vi "字符串案例之字符串公式解析(下).vi"() -> ()   [LabVIEW 2018]
panel:
  out "数组 5":dbl[](array[numeric])
  out "数组 4":dbl[](array[numeric])
  out "数组 3":string[](array[string])
  out "数组 2":string[](array[string])
  out "数组":dbl[](array[numeric])
  in  "字符串":string
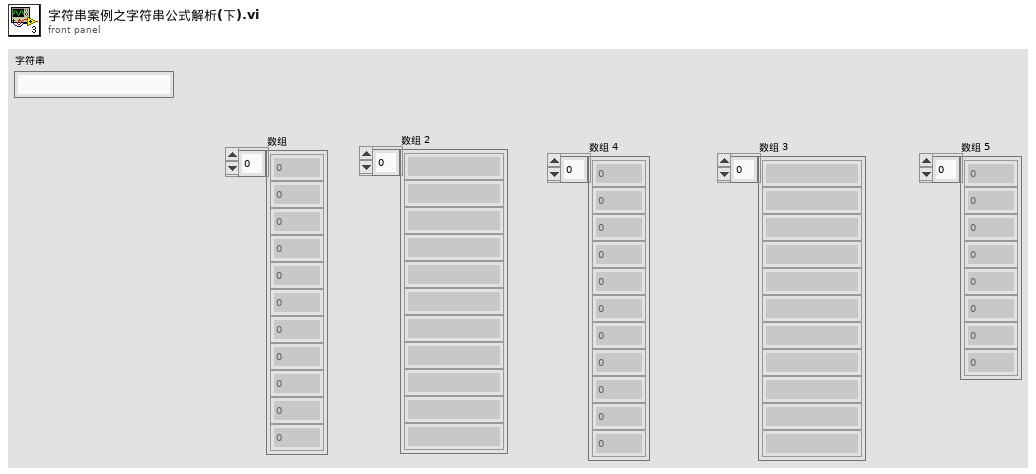
[diagram p1: front panel]
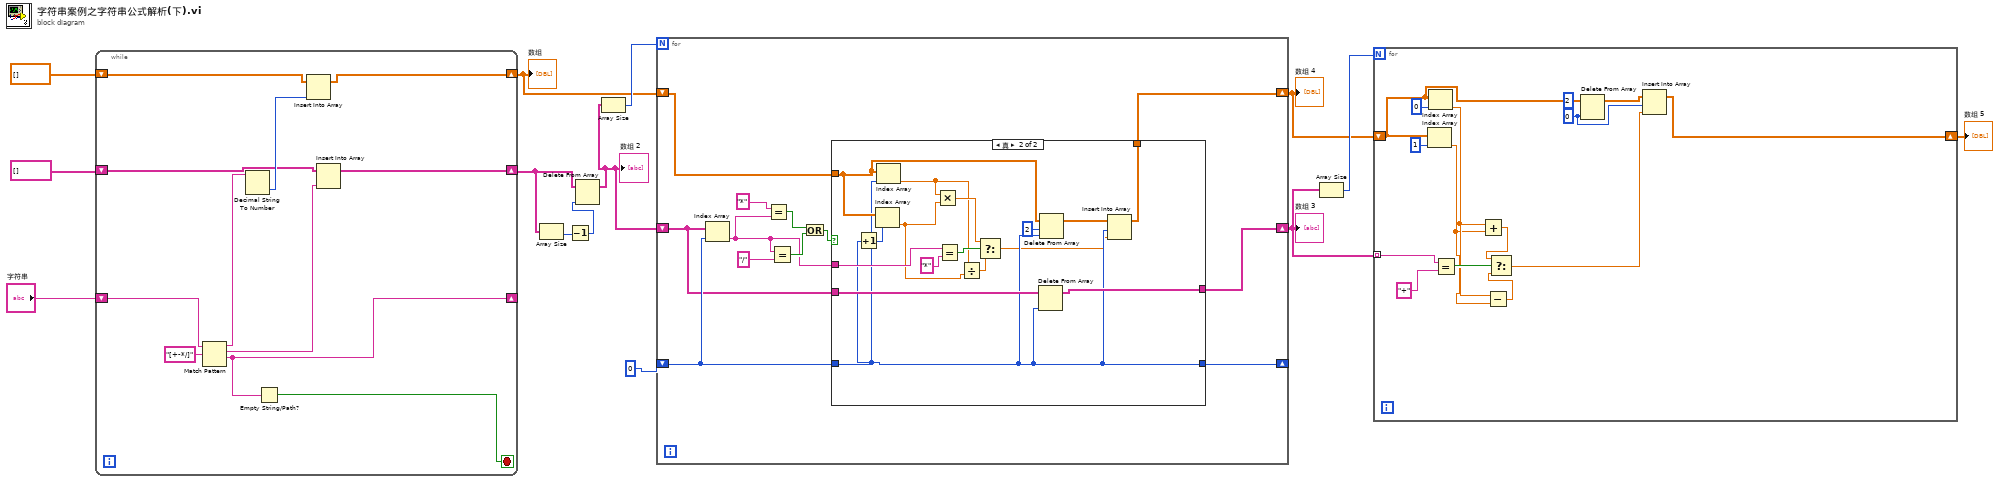
[diagram p0: block diagram]
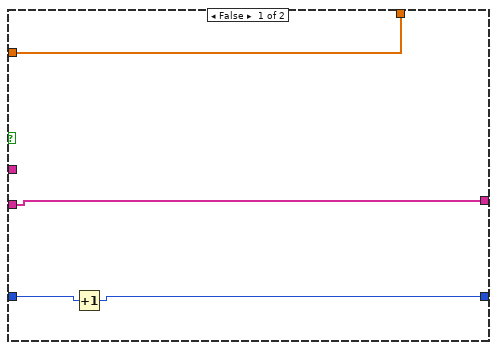
[diagram p2: hidden frame]
diagram:
  n1 = while {
    shift-right: [w20] -> w5
    shift-left: dbl[] [] -> [w21]
    shift-right: [w17] -> w11
    shift-left: string[] [] -> [w18]
    shift-right: [w16] -> _
    shift-left: "字符串" -> [w24]
    stop <- w15 stop-if-true
    n2 = Match Pattern(string=w24, regular expression="[+-*/]" ("正则表达式")) -> (before substring=w23:string, match substring=w19:string, after substring=w16:string)  [unwired: 1 in, 1 out]
    n3 = Decimal String To Number(string=w23) -> (number=w22:i32)  [unwired: 2 in, 1 out]
    n4 = Empty String/Path?(string/path=w16) -> (empty?=w15:bool)
    n5 = Insert Into Array(array=w21, new element=w22) -> (w20:dbl[])  [unwired: 1 in]
    n6 = Insert Into Array(array=w18, new element=w19) -> (w17:string[])  [unwired: 1 in]
  }
  "数组" <- w5
  n7 = Array Size(array=w11) -> (size(s)=w10:i32)
  n8 = Decrement(x=w10) -> (x-1=w9:i32)
  n9 = Delete From Array(array=w11, index=w9) -> (array with subset deleted=w7:string[])  [unwired: 1 in, 1 out]
  "数组 2" <- w7
  n10 = Array Size(array=w7) -> (size(s)=w8:i32)
  n11 = for {
    N: w8 -> [_]
    shift-right: [w32] -> _
    shift-left: 0 -> [w31]
    shift-right: [w29] -> w3
    shift-left: w7 -> [w30]
    shift-right: [w26] -> w2
    shift-left: w5 -> [w28]
    n12 = Index Array(array=w30, index=w31) -> (element=w27:string)
    n13 = Equal?(x="*", y=w27) -> (x = y?=w34:bool)
    n14 = Equal?(x=w27, y="/") -> (x = y?=w35:bool)
    n15 = Or(x=w34, y=w35) -> (x .or. y?=w33:bool)
    n16 = case shown="真" w33 {
      tunnel: w31 -> [w41 w44]
      tunnel: [w40 w44] -> w32
      tunnel: w30 -> [w39 w57]
      tunnel: [w39 w56] -> w29
      tunnel: w28 -> [w38 w47]
      tunnel: w27 -> [_ w53]
      tunnel: [w38 w42] -> w26
      frame False {
        n17 = Increment(x=w41) -> (x+1=w40:i32)
      }
      frame True {
        n18 = Increment(x=w44) -> (x+1=w55:i32)
        n19 = Index Array(array=w47, index=w55) -> (element=w48:dbl)
        n20 = Index Array(array=w47, index=w44) -> (element=w49:dbl)
        n21 = Multiply(x=w49, y=w48) -> (x*y=w51:dbl)
        n22 = Equal?(x=w53, y="*") -> (x = y?=w52:bool)
        n23 = Divide(x=w49, y=w48) -> (x/y=w50:dbl)
        n24 = Select(t=w51, s=w52, f=w50) -> (s? t:f=w43:dbl)
        n25 = Delete From Array(array=w57, index=w44) -> (array with subset deleted=w56:string[])  [unwired: 1 in, 1 out]
        n26 = Delete From Array(array=w47, length=2 ("长度"), index=w44) -> (array with subset deleted=w45:dbl[])  [unwired: 1 out]
        n27 = Insert Into Array(array=w45, index=w44, new element=w43) -> (w42:dbl[])
      }
    }
  }
  "数组 3" <- w3
  "数组 4" <- w2
  n28 = Array Size(array=w3) -> (size(s)=w4:i32)
  n29 = for {
    N: w4 -> [_]
    tunnel: w3 -> [w71] mode=indexing
    shift-right: [w58] -> w1
    shift-left: w2 -> [w63]
    w59 = 0 ("索引")
    n30 = Index Array(array=w63, index=1 ("索引")) -> (element=w64:dbl)
    n31 = Index Array(array=w63, index=0 ("索引")) -> (element=w65:dbl)
    n32 = Equal?(x=w71, y="+") -> (x = y?=w70:bool)
    n33 = Add(x=w65, y=w64) -> (x+y=w69:dbl)
    n34 = Subtract(x=w65, y=w64) -> (x-y=w68:dbl)
    n35 = Select(t=w69, s=w70, f=w68) -> (s? t:f=w60:dbl)
    n36 = Delete From Array(array=w63, length=2 ("长度"), index=w59) -> (array with subset deleted=w61:dbl[])  [unwired: 1 out]
    n37 = Insert Into Array(array=w61, index=w59, new element=w60) -> (w58:dbl[])
  }
  "数组 5" <- w1
